vi "Data.vi"(8 "error in (no error)":errorcluster, 10 "Channels (All)":string[](array[string]), 11 "Group Buffer DBL in":refnum<class "Group Buffer DBL.lvclass">) -> (0 "error out":errorcluster, 2 "Group Data":T1, 3 "Group Buffer DBL out":refnum<class "Group Buffer DBL.lvclass">)   [LabVIEW 2020, in "VolatusHistorian.lvlib" / "Group Buffer DBL.lvclass"]
uses:
  Group Buffer DBL.lvclass
  Group Data.ctl
  Channel Data.ctl
  Group Buffer DBL.lvclass/Group Buffer DBL.ctl
  Channel Buffer DBL/Channel Buffer DBL.lvclass/Channel Buffer DBL.ctl
  Channel Buffer DBL/Name.vi
  Channel Buffer DBL/Channel Buffer DBL.lvclass
  VolatusHistorian.lvlib
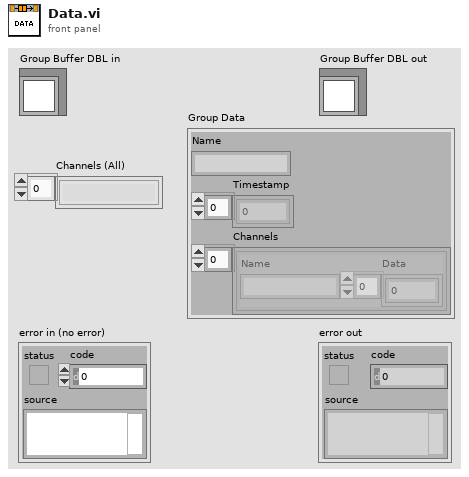
[diagram p1: front panel]
types:
  T1 = typedef "VolatusHistorian.lvlib/Group Data.ctl" = cluster{"Name":string, "Timestamp":dbl[], "Channels":T2[]}
  T2 = typedef "VolatusHistorian.lvlib/Channel Data.ctl" = cluster{"Name":string, "Data":dbl[]}
  T3 = typedef "VolatusHistorian.lvlib/Group Buffer DBL.lvclass/Ref.ctl" = cluster{"Time":refnum<queue>, "Channel Name Map":map{string, i32}, "Group Info":T4, "Channels":refnum<class "Channel Buffer DBL.lvclass">[], "Channel Names":string[]}
  T4 = typedef "VectoConfig.lvlib/Group Info.ctl" = cluster{"System":string, "Cluster":string, "Node":string, "Task":string, "Name":string}
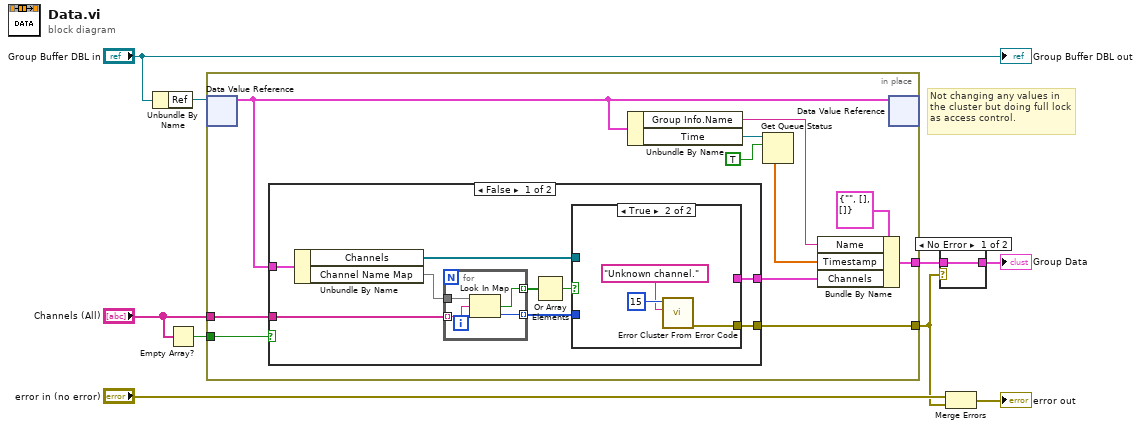
[diagram p0: block diagram]
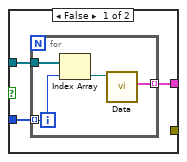
[diagram p3: hidden frame]
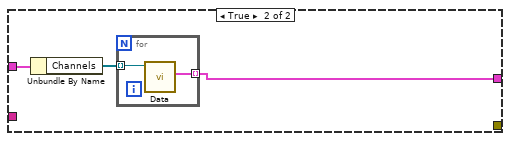
[diagram p4: hidden frame]
diagram:
  # "Not changing any values in the cluster but doing full lock as access control."
  n1 = Unbundle By Name("Group Buffer DBL in") -> ("Ref"=w7:refnum<data-value>)
  n2 = Empty Array?(array="Channels (All)") -> (empty?=w5:bool)
  n3 = in-place {
    in-place-border: "Channels (All)" -> [w19]
    in-place-border: w5 -> [w20]
    in-place-border: [w11] -> w3
    in-place-border: [w10] -> w1
    n4 = in-place-dvr #1(w7) -> (w18:T3)  [unwired: 1 out]
    n5 = case shown="False" w20 {
      tunnel: w18 -> [w29 w46]
      tunnel: w19 -> [w27 _]
      tunnel: [w22 w44] -> w12
      tunnel: [w21 _] -> w10
      frame False {
        n6 = Unbundle By Name(w29) -> ("Channels"=w23:refnum<class "Channel Buffer DBL.lvclass">[], "Channel Name Map"=w28:map{string, i32})
        n7 = for {
          tunnel: w28 -> [w43]
          tunnel: w27 -> [w42] mode=indexing
          tunnel: [w41] -> w24 mode=indexing
          tunnel: [w40] -> w26 mode=indexing
          n8 = Look In Map(map=w43, key=w42) -> (key not found?=w40:bool, value=w41:i32)  [unwired: 1 in]
        }
        n9 = Or Array Elements(Boolean array=w26) -> (logical OR=w25:bool)
        n10 = case shown="True" w25 {
          tunnel: w24 -> [w32 _]
          tunnel: w23 -> [w31 _]
          tunnel: [w30 _] -> w22
          tunnel: [_ w37] -> w21
          frame False {
            n11 = for {
              tunnel: w32 -> [w35] mode=indexing
              tunnel: w31 -> [w36]
              tunnel: [w33] -> w30 mode=indexing
              n12 = Index Array(array=w36, index=w35) -> (element=w34:refnum<class "Channel Buffer DBL.lvclass">)
              n13 = call "Data.vi"("Channel Buffer DBL in"=w34) -> ("Channel Data"=w33:T2)  [unwired: 8 in, 2 out]
            }
          }
          frame True {
            n14 = call <vilib>:"Error Cluster From Error Code.vi"("error message (\"\")"="Unknown channel.", "error code (0)"=15) -> ("error out"=w37:errorcluster)  [unwired: 7 in]
          }
        }
      }
      frame True {
        n15 = Unbundle By Name(w46) -> ("Channels"=w45:refnum<class "Channel Buffer DBL.lvclass">[])
        n16 = for {
          tunnel: w45 -> [w48] mode=indexing
          tunnel: [w47] -> w44 mode=indexing
          n17 = call "Data.vi"("Channel Buffer DBL in"=w48) -> ("Channel Data"=w47:T2)  [unwired: 8 in, 2 out]
        }
      }
    }
    n18 = Unbundle By Name(w18) -> ("Group Info.Name"=w14:string, "Time"=w17:refnum<queue>)
    n19 = Get Queue Status(queue=w17, return elements? (F)=TRUE) -> (elements=w13:dbl[])  [unwired: 1 in, 7 out]
    n20 = Bundle By Name(cluster=T1 {"Name"="", "Timestamp"=[], "Channels"=[]} ("Group Data"), "Name"=w14, "Timestamp"=w13, "Channels"=w12) -> (w11:T1)
    n21 = in-place-dvr #1(w18) -> ()  [unwired: 2 out]
  }
  n22 = case shown="No Error" w1 {
    tunnel: [w49 _] -> w4
    tunnel: w3 -> [w49 _]
    frame No Error {
    }
    frame Error {
    }
  }
  "Group Data" <- w4
  n23 = Merge Errors("error in (no error)", w1) -> (→"error out":errorcluster)
  "Group Buffer DBL out" <- "Group Buffer DBL in"
